vi "Queue Receiver.vi"() -> ()   [LabVIEW 2009]
uses:
  <vilib>/Platform/TimedLoop/XDataNode/XDataNode.xnode
  <vilib>/Platform/TimedLoop/XDataNode/loadlvalarms.vi
  <vilib>/Platform/TimedLoop/XDataNode/timing_clust.ctl
  <vilib>/Platform/TimedLoop/XDataNode/nitl_modes.ctl
  <vilib>/Platform/TimedLoop/XDataNode/wakeup.ctl
  <vilib>/Platform/TimedLoop/XDataNode/XDNodeRunTimeDep.lvlib
panel:
  out "element":T1
  in  "OK Button":bool
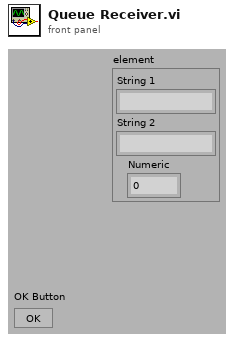
[diagram p1: front panel]
types:
  T1 = cluster{"String 1":string, "String 2":string, "Numeric":dbl}
  T2 = typedef "XDNodeRunTimeDep.lvlib/timing_clust.ctl" = cluster{"Expected End [f-1]":u64, "Actual End [f-1]":u64, "Finished Late? [f-1]":bool, "Expected End [i-1]":u64, "Actual End [i-1]":u64, "Finished Late? [i-1]":bool, "Expected Start [i]":u64, "Actual Start [i]":u64, "Expected Start [f]":u64, "Actual Start [f]":u64, "Source Name":string, "Structure Name":string, "Period":i64, "Deadline":i64, "Offset":i64, "Start":i64, "Priority":i32, "Timeout":i32, "Mode":T3, "Wakeup Reason":T4, "Error":errorcluster, "Source Type":string, "Secondary Source Type":string, "Global End Time":u64, "Global Start Time":u64, "Frame Duration":u64, "Iteration Duration":u64, "Assigned CPU":i32, "I/O Scan Engine Mode":u32}
  T3 = typedef "XDNodeRunTimeDep.lvlib/nitl_modes.ctl" = enum32{"No Change", "Process missed periods, maintain original phase", "Discard missed periods, maintain original phase", "Process missed periods, ignore original phase", "Discard missed periods, ignore original phase"}
  T4 = typedef "XDNodeRunTimeDep.lvlib/wakeup.ctl" = enum32{"Normal", "Aborted", "Asynchronous wakeup", "Timing source error", "Timed loop error", "Timeout"}
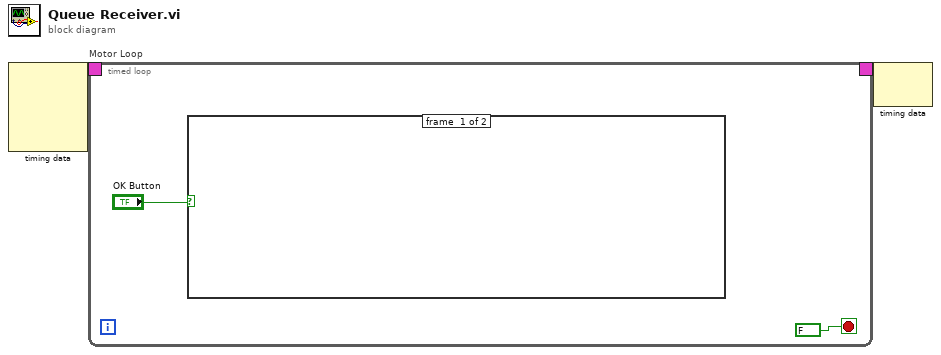
[diagram p0: block diagram]
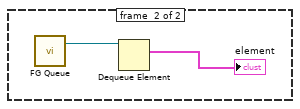
[diagram p2: hidden frame]
diagram:
  n1 = node-c288() -> (w2:T2)  [unwired: 4 in]
  n2 = timed-loop "Motor Loop" {
    timing: w2 -> [_]
    timing-out: [_] -> w1
    stop <- FALSE stop-if-true
    n3 = case shown="True" "OK Button" {
      frame #0 {
      }
      frame #1 {
        n4 = call "FG Queue.vi"() -> ("queue out"=w6:refnum<queue>)  [unwired: 3 in]
        n5 = Dequeue Element(queue=w6) -> (element=→"element":T1)  [unwired: 2 in, 3 out]
      }
    }
  }
  n6 = node-c288(w1) -> ()  [unwired: 1 out]
